vi "Module Timeout--constant.vi"() -> (3 "Module Timeout":i32)   [LabVIEW 2017, in "MQTT.lvlib"]
doc: "A module-wide common value to use as the timeout for various synchronization actions.\n_____\nBased on Delacor QMH Project Template 3.1.0.34."
uses:
  MQTT.lvlib
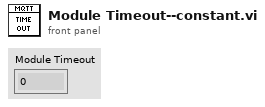
[diagram p1: front panel]
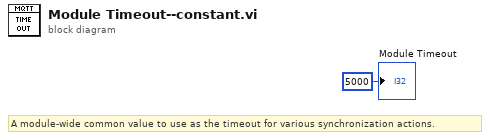
[diagram p0: block diagram]
diagram:
  # "A module-wide common value to use as the timeout for various synchronization actions."
  "Module Timeout" <- 5000 ("Module Timeout")
